vi "Stop Global Variable.vi"() -> ()   [LabVIEW 2020]
panel:
  in  "Stop":bool
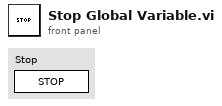
[diagram p1: front panel]
diagram:
